vi "Get Result.vi"(4 "Controller name":string, 6 "Last request":bool, 8 "error in (no error)":errorcluster, 11 "Instrument Recorder in":refnum<class "Lockin Digitizer.lvclass">) -> (0 "error out":errorcluster, 2 "Result":refnum<class "Acquired Result.lvclass">, 3 "Instrument Recorder out":refnum<class "Lockin Digitizer.lvclass">)   [LabVIEW 2021, in "Lockin Digitizer.lvclass"]
uses:
  Lockin Digitizer.lvclass
  Lockin Digitizer.lvclass/Lockin Digitizer.ctl
  Pulse Recorder Actor/Pulse Recorder Actor.lvclass
  NHMFL_Core/Libraries/Instruments/Results/Acquired Result/Acquired Result.lvclass
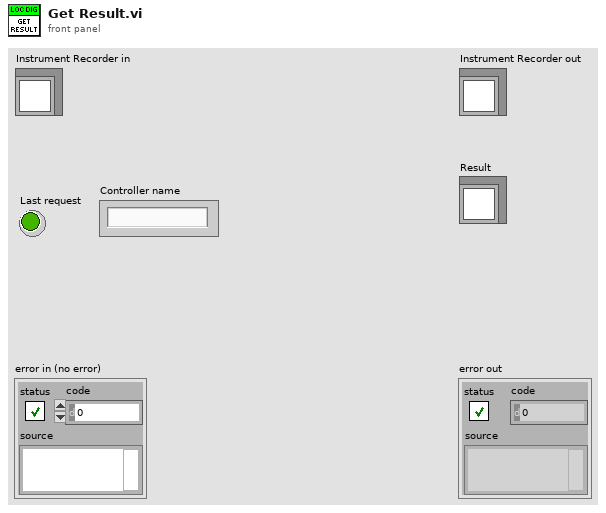
[diagram p1: front panel]
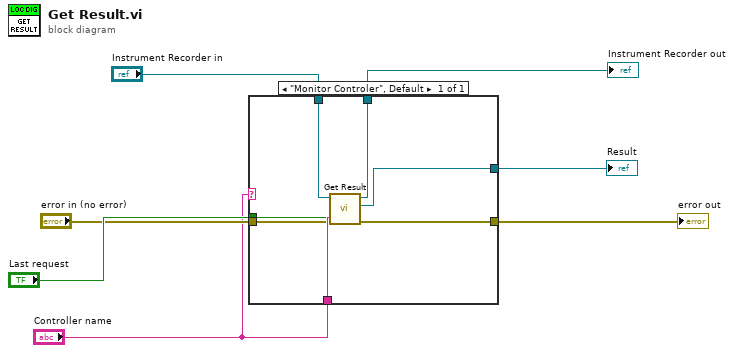
[diagram p0: block diagram]
diagram:
  n1 = case shown="\"Monitor Controler\", Default" "Controller name" {
    tunnel: [w14] -> w7
    tunnel: [w13] -> w6
    tunnel: [w12] -> w5
    tunnel: "Controller name" -> [w11]
    tunnel: "Last request" -> [w10]
    tunnel: "error in (no error)" -> [w9]
    tunnel: "Instrument Recorder in" -> [w8]
    frame "Monitor Controler", Default {
      n2 = call-parent "Get Result.vi"("Controller name"=w11, "Last request"=w10, "error in (no error)"=w9, "Instrument Recorder in"=w8) -> ("error out"=w14:errorcluster, "Result"=w13:refnum<class "Acquired Result.lvclass">, "Instrument Recorder out"=w12:refnum<class "Lockin Digitizer.lvclass">)  [unwired: 5 in]
    }
  }
  "error out" <- w7
  "Instrument Recorder out" <- w5
  "Result" <- w6
